vi "Write_parameter.vi"(8 "error in (no error)":errorcluster caption="entrée d'erreur (pas d'erreur)", 10 "Parameter":string, 11 "Class Instrument Multimeter en entrée":refnum<class "Class Instrument Spectrum_Analyser.lvclass">) -> (0 "error out":errorcluster caption="sortie d'erreur", 3 "Class Instrument Multimeter en sortie":refnum<class "Class Instrument Spectrum_Analyser.lvclass">)   [LabVIEW 2020, in "Library Instrument & Equipement.lvlib" / "Library Instruments.lvlib" / "Class Instrument Spectrum_Analyser.lvclass"]
uses:
  Class Instrument Spectrum_Analyser.lvclass
  Commun VI/TypeDef/Command Spectrum_Analyser/Parameter Spectrum_Analyser.ctl
  Spectrum Analyser/Class Spectrum Analyser (Default)/Class Spectrum Analyser (Default).lvclass
  JSON API/JSON Value/Set from JSON string.vi
  Instrument (Default)/Class Instrument (Default).lvclass
  JSON API/JSON Value/JSON Value.lvclass
  Class Instrument Spectrum_Analyser.lvclass/Class Instrument Spectrum_Analyser.ctl
  JSON API/Variant JSON/Variant JSON.lvlib
  JSON API/Get Polymorphic/JSON GetSet.lvlib
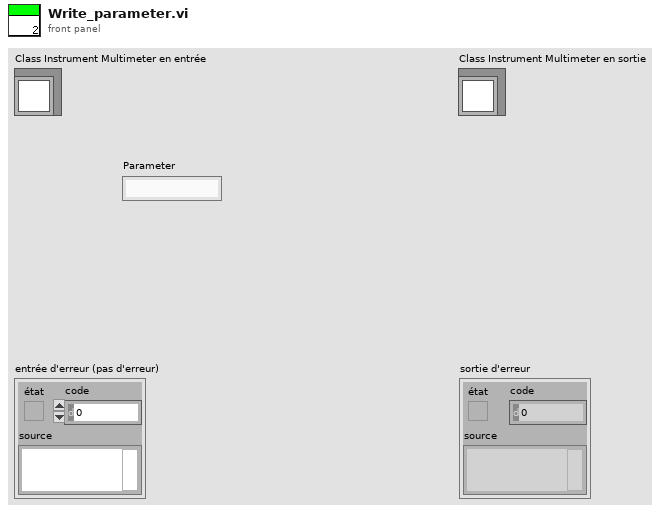
[diagram p1: front panel]
types:
  T1 = typedef "Parameter Spectrum_Analyser.ctl" = cluster{"Device @":string, "Class Spectrum Analyser":refnum<class "Class Spectrum Analyser (Default).lvclass">, "Center Freq (MHz)":dbl, "Freq Span (MHz)":dbl, "Ref Level (dBm)":dbl, "Threshold (dBm)":dbl, "TimeOut":i16}
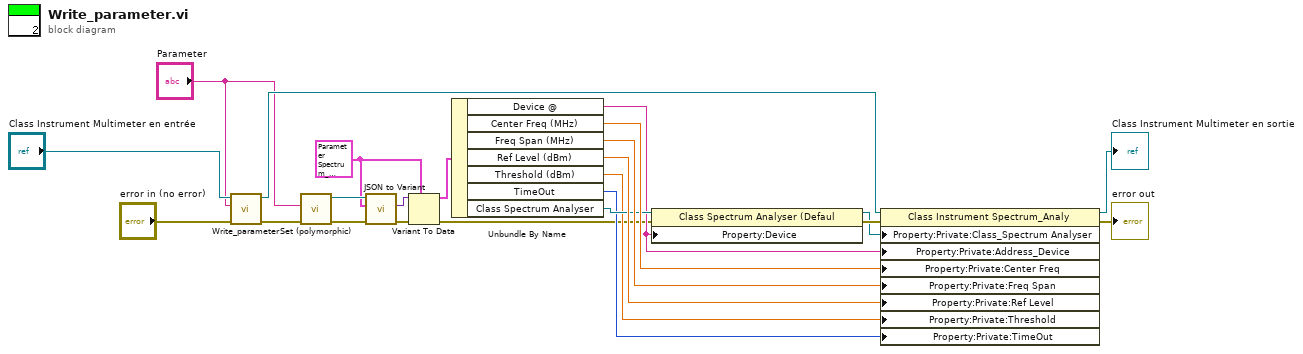
[diagram p0: block diagram]
diagram:
  w7 = T1 {"Device @"="", "Class Spectrum Analyser"=refnum, "Center Freq (MHz)"=0.0, "Freq Span (MHz)"=0.0, "Ref Level (dBm)"=0.0, "Threshold (dBm)"=0.0, "TimeOut"=0} ("Parameter")
  n1 = call-parent "Write_parameter.vi"("error in (no error)"="error in (no error)", "Parameter"="Parameter", "Class Instrument (Default) en entrée"="Class Instrument Multimeter en entrée") -> ("error out"=w11:errorcluster, "Class Instrument (Default) en sortie"=w10:refnum<class "Class Instrument Spectrum_Analyser.lvclass">)  [unwired: 7 in]
  n2 = call-poly "Set (polymorphic).vi"("error in (no error)"=w11, "JSON stream"="Parameter") -> ("error out"=w21:errorcluster, "JSON Value out"=w23:refnum<class "JSON Value.lvclass">)  [unwired: 7 in, 1 out]
  n3 = call "JSON to Variant.vi"("error in (no error)"=w21, "Variant (Data Type)"=w7, "JSON Value"=w23) -> ("error out"=w22:errorcluster, "Variant out"=w20:variant)  [unwired: 7 in]
  n4 = Variant To Data(error in=w22, type=w7, Variant=w20) -> (data=w17:T1, error out=w2:errorcluster)
  n5 = Unbundle By Name(w17) -> ("Device @"=w4:string, "Center Freq (MHz)"=w14:dbl, "Freq Span (MHz)"=w15:dbl, "Ref Level (dBm)"=w16:dbl, "Threshold (dBm)"=w5:dbl, "TimeOut"=w6:i16, "Class Spectrum Analyser"=w13:refnum<class "Class Spectrum Analyser (Default).lvclass">)
  n6 = property class="Class Spectrum Analyser (Defaul"(reference=w13, error in=w2, "Property:Device"=w4) -> (reference out=w1:refnum<class "Class Spectrum Analyser (Default).lvclass">, error out=w3:errorcluster)
  n7 = property class="Class Instrument Spectrum_Analy"(reference=w10, error in=w3, "Property:Private:Class_Spectrum Analyser"=w1, "Property:Private:Address_Device"=w4, "Property:Private:Center Freq"=w14, "Property:Private:Freq Span"=w15, "Property:Private:Ref Level"=w16, "Property:Private:Threshold"=w5, "Property:Private:TimeOut"=w6) -> (reference out=→"Class Instrument Multimeter en sortie":refnum<class "Class Instrument Spectrum_Analyser.lvclass">, error out=→"error out":errorcluster)
